vi "总磷总氮XML解析.vi"(10 "启动模式":enum16{"水样测量", "零液测量", "标液测量"}(ring), 11 "启动参数":enum16{"总磷", "总氮", "总磷海水", "总氮海水"}(ring)) -> (2 "步骤时间":string[](array[string]), 3 "步骤名":string[](array[string]))   [LabVIEW 2016]
uses:
  <vilib>/Utility/sysdir.llb/System Directory Type.ctl
  <vilib>/xml/Load XML File.vi
  <vilib>/xml/Close Reference(Node).vi
  <resource>/objmgr/DOMUserDefRef.rc
  <vilib>/xml/NI_XML.lvlib
panel:
  out "添加的路径":path
  out "XML字符串":string="<?xml version=\"1.0\" encoding=\"ISO-8859-1\"?>\n<bookstore>\n<book ISBN=\"978-0545128285\">\n  <title lang=\"en\">The Tales of Beedle the Bard</title>\n  <author>J. K. Rowling</author>\n  <year>2008</year>\n  <price>12.99</price>\n</book>\n<book ISBN=\"978-0316160209\">\n  <title lang=\"en\">Eclipse</title>\n  <author>Stephenie Meyer</author>\n  <year>2007</year>\n  <price>19.99</price>\n</book>\n<book ISBN=\"978-0316067928\">\n  <title lang=\"en\">Breaking Dawn</title>\n  <author>Stephenie Meyer</author>\n  <year>2008</year>\n  <price>22.99</price>\n</book>\n<book ISBN=\"978-0316017923\">\n  <title lang=\"en\">Outliers: The Story of Success</title>\n  <author>Malcolm Gladwell</author>\n  <year>2008</year>\n  <price>27.99</price>\n</book>\n<book ISBN=\"978-0596007645\">\n  <title lang=\"en\">XML in a Nutshell</title>\n  <author>Elliotte Rusty Harold</author>\n  <author>W. Scott Means</author>\n  <year>2004</year>\n  <price>39.95</price>\n</book>\n</bookstore>"
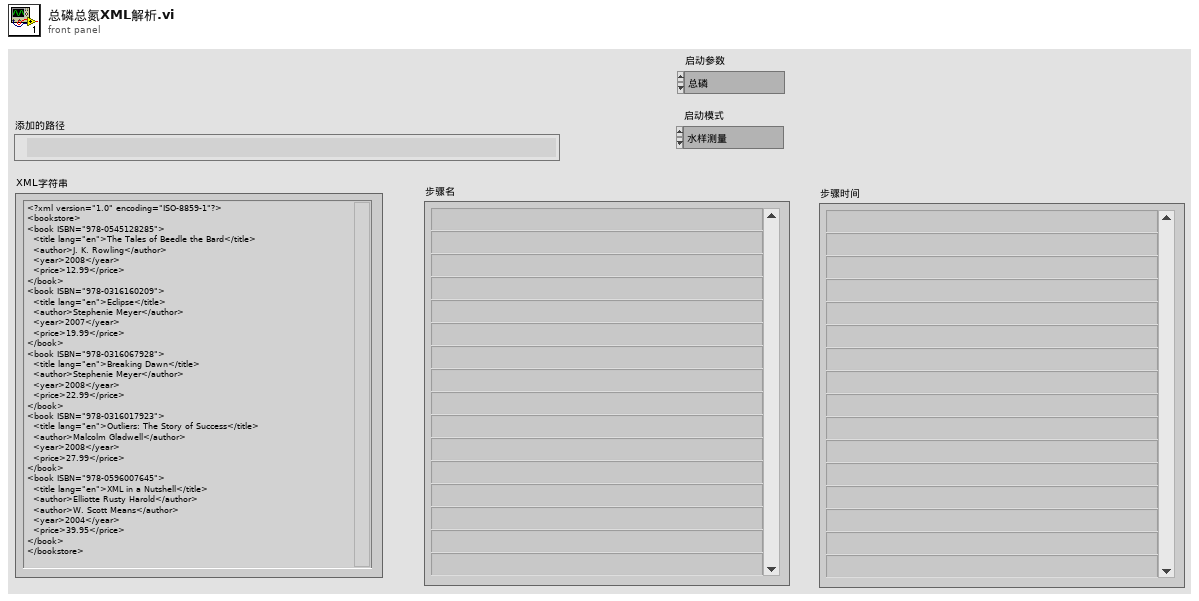
[diagram p1: front panel]
types:
  T1 = typedef "System Directory Type.ctl" = i32
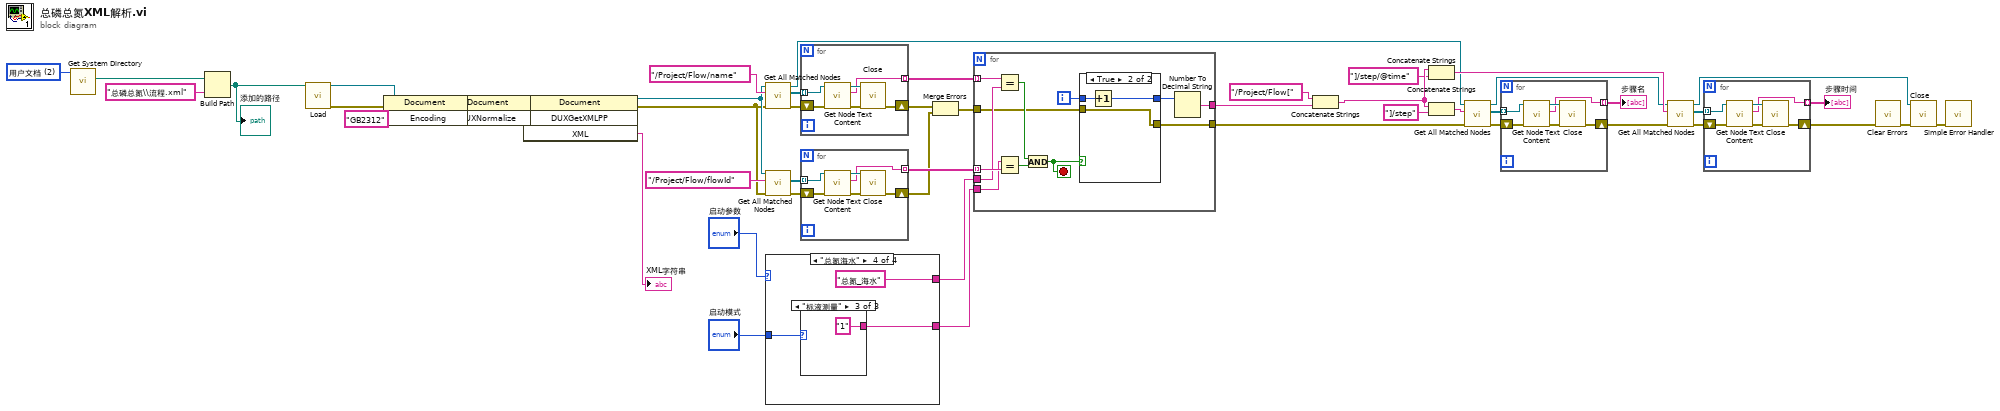
[diagram p0: block diagram]
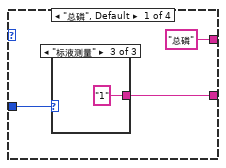
[diagram p2: hidden frame]
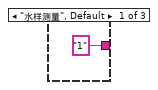
[diagram p3: hidden frame]
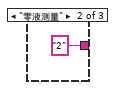
[diagram p4: hidden frame]
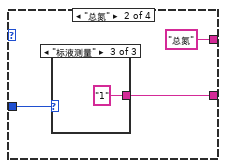
[diagram p5: hidden frame]
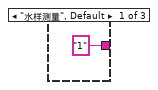
[diagram p6: hidden frame]
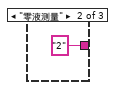
[diagram p7: hidden frame]
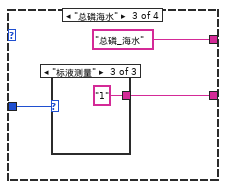
[diagram p8: hidden frame]
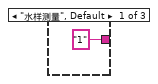
[diagram p9: hidden frame]
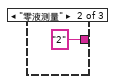
[diagram p10: hidden frame]
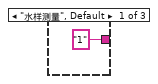
[diagram p11: hidden frame]
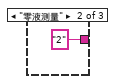
[diagram p12: hidden frame]
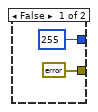
[diagram p13: hidden frame]
diagram:
  w27 = T1 2 items=["用户目录"=0, "用户桌面"=1, "用户文档"=2, "用户应用程序数据"=3, "用户设置"=4, "用户临时目录"=5, "公共文档"=6, "公共应用程序数据"=7, "公共设置"=8, "公共缓存"=13, "系统核心库"=9, "系统安装库"=10, "应用程序文件"=11, "启动盘根目录"=12] ("system directory type")
  n1 = call <vilib>:"Get System Directory.vi"("system directory type"=w27) -> ("system directory"=w26:path)  [unwired: 10 in]
  n2 = Build Path(base path=w26, name or relative path="总磷总氮\\流程.xml" ("名称或相对路径")) -> (appended path=w24:path)
  "添加的路径" <- w24
  n3 = call-poly <vilib>:"Load.vi"("path to XML document"=w24) -> ("DOM document out"=w47:refnum<k20>, "error out"=w46:errorcluster)  [unwired: 12 in, 1 out]
  n4 = property on="属性节点" class="Document"(reference=w47, error in=w46, "Encoding"="GB2312" ("文档编码")) -> (reference out=w44:refnum<k20>, error out=w43:errorcluster)
  n5 = invoke on="Invoke Node" class="Document" method="DUXNormalize"(reference=w44, error in=w43) -> (reference out=w41:refnum<k20>, error out=w42:errorcluster)  [unwired: 1 in, 1 out]
  n6 = invoke on="Invoke Node" class="Document" method="DUXGetXMLPP"(reference=w41, error in=w42) -> (reference out=w17:refnum<k20>, error out=w16:errorcluster, "XML"=→"XML字符串":string)  [unwired: 2 in, 1 out]
  n7 = call <vilib>:"Get All Matched Nodes.vi"("error in (no error)"=w16, "XPath expression"="/Project/Flow/name", "node in"=w17) -> ("error out"=w13:errorcluster, "node result array"=w22:refnum<k20>[], "node out"=w14:refnum<k20>)  [unwired: 6 out]
  n8 = call <vilib>:"Get All Matched Nodes.vi"("error in (no error)"=w16, "XPath expression"="/Project/Flow/flowId", "node in"=w17) -> ("error out"=w12:errorcluster, "node result array"=w20:refnum<k20>[])  [unwired: 7 out]
  n9 = case shown="\"总氮海水\"" "启动参数" {
    tunnel: "启动模式" -> [w53 w59 w65 w71]
    tunnel: ["总磷" "总氮" "总磷_海水" "总氮_海水"] -> w2
    tunnel: [w51 w57 w64 w69] -> w1
    frame "总磷", Default {
      n10 = case shown="\"标液测量\"" w53 {
        tunnel: ["1" "2" "1"] -> w51
        frame "水样测量", Default {
        }
        frame "零液测量" {
        }
        frame "标液测量" {
        }
      }
    }
    frame "总氮" {
      n11 = case shown="\"标液测量\"" w59 {
        tunnel: ["1" "2" "1"] -> w57
        frame "水样测量", Default {
        }
        frame "零液测量" {
        }
        frame "标液测量" {
        }
      }
    }
    frame "总磷海水" {
      n12 = case shown="\"标液测量\"" w65 {
        tunnel: ["1" "2" "1"] -> w64
        frame "水样测量", Default {
        }
        frame "零液测量" {
        }
        frame "标液测量" {
        }
      }
    }
    frame "总氮海水" {
      n13 = case shown="\"标液测量\"" w71 {
        tunnel: ["1" "2" "1"] -> w69
        frame "水样测量", Default {
        }
        frame "零液测量" {
        }
        frame "标液测量" {
        }
      }
    }
  }
  n14 = for {
    tunnel: w22 -> [w79] mode=indexing
    shift-right: [w80] -> w10
    shift-left: w13 -> [w78]
    tunnel: [w75] -> w21 mode=indexing
    n15 = call <vilib>:"Get Node Text Content.vi"("error in (no error)"=w78, "node in"=w79) -> ("error out"=w76:errorcluster, "node text"=w75:string, "node out"=w77:refnum<k20>)  [unwired: 7 in]
    n16 = call-poly <vilib>:"Close.vi"("error in (no error)"=w76, "node"=w77) -> ("error out"=w80:errorcluster)  [unwired: 7 out]
  }
  n17 = for {
    shift-right: [w86] -> w11
    shift-left: w12 -> [w85]
    tunnel: [w82] -> w18 mode=indexing
    tunnel: w20 -> [w81] mode=indexing
    n18 = call <vilib>:"Get Node Text Content.vi"("error in (no error)"=w85, "node in"=w81) -> ("error out"=w83:errorcluster, "node text"=w82:string, "node out"=w84:refnum<k20>)  [unwired: 7 in]
    n19 = call-poly <vilib>:"Close.vi"("error in (no error)"=w83, "node"=w84) -> ("error out"=w86:errorcluster)  [unwired: 7 out]
  }
  n20 = Merge Errors(w10, w11) -> (w9:errorcluster)
  n21 = for {
    tunnel: w21 -> [w98] mode=indexing
    tunnel: w18 -> [w97] mode=indexing
    tunnel: [w91] -> w15
    tunnel: w2 -> [w90]
    tunnel: w1 -> [w89]
    tunnel: w9 -> [w88]
    tunnel: [w87] -> w8
    i -> [w93]
    stop <- w94 stop-if-true
    n22 = Equal?(x=w98, y=w90) -> (x = y?=w95:bool)
    n23 = Equal?(x=w89, y=w97) -> (x = y?=w96:bool)
    n24 = And(x=w95, y=w96) -> (x .and. y?=w94:bool)
    n25 = case shown="True" w94 {
      tunnel: w93 -> [_ w102]
      tunnel: [255 w101] -> w92
      tunnel: w88 -> [_ w103]
      tunnel: [errorcluster {"status"=TRUE, "code"=0, "source"=""} ("错误常量") w103] -> w87
      frame False {
      }
      frame True {
        n26 = Increment(x=w102) -> (x+1=w101:i32)
      }
    }
    n27 = Number To Decimal String(number=w92) -> (decimal integer string=w91:string)  [unwired: 1 in]
  }
  n28 = Concatenate Strings("/Project/Flow[" ("XPath expression"), w15) -> (w34:string)
  n29 = Concatenate Strings(w34, "]/step/@time" ("XPath expression")) -> (w32:string)
  n30 = Concatenate Strings(w34, "]/step" ("XPath expression")) -> (w35:string)
  n31 = call <vilib>:"Get All Matched Nodes.vi"("error in (no error)"=w8, "XPath expression"=w35, "node in"=w14) -> ("error out"=w50:errorcluster, "node result array"=w45:refnum<k20>[], "node out"=w30:refnum<k20>)  [unwired: 6 out]
  n32 = for {
    tunnel: w45 -> [w108] mode=indexing
    shift-right: [w109] -> w38
    shift-left: w50 -> [w107]
    tunnel: [w104] -> w40 mode=indexing
    n33 = call <vilib>:"Get Node Text Content.vi"("error in (no error)"=w107, "node in"=w108) -> ("error out"=w105:errorcluster, "node text"=w104:string, "node out"=w106:refnum<k20>)  [unwired: 7 in]
    n34 = call-poly <vilib>:"Close.vi"("error in (no error)"=w105, "node"=w106) -> ("error out"=w109:errorcluster)  [unwired: 7 out]
  }
  "步骤名" <- w40
  n35 = call <vilib>:"Get All Matched Nodes.vi"("error in (no error)"=w38, "XPath expression"=w32, "node in"=w30) -> ("error out"=w37:errorcluster, "node result array"=w31:refnum<k20>[], "node out"=w29:refnum<k20>)  [unwired: 6 out]
  n36 = for {
    tunnel: w31 -> [w114] mode=indexing
    shift-right: [w115] -> w6
    shift-left: w37 -> [w113]
    tunnel: [w110] -> w28 mode=indexing
    n37 = call <vilib>:"Get Node Text Content.vi"("error in (no error)"=w113, "node in"=w114) -> ("error out"=w111:errorcluster, "node text"=w110:string, "node out"=w112:refnum<k20>)  [unwired: 7 in]
    n38 = call-poly <vilib>:"Close.vi"("error in (no error)"=w111, "node"=w112) -> ("error out"=w115:errorcluster)  [unwired: 7 out]
  }
  "步骤时间" <- w28
  n39 = call <vilib>:"Clear Errors.vi"("error in (no error)"=w6) -> ("error out"=w5:errorcluster)  [unwired: 5 in, 1 out]
  n40 = call-poly <vilib>:"Close.vi"("error in (no error)"=w5, "node"=w29) -> ("error out"=w7:errorcluster)  [unwired: 7 out]
  n41 = call <vilib>:"Simple Error Handler.vi"("error in (no error)"=w7) -> ()  [unwired: 4 in, 5 out]
